vi "Get Travel Reading.vi"(8 "error in (no error)":errorcluster, 11 "ESM303 in":refnum<class "ESM303.lvclass">) -> (0 "error out":errorcluster, 2 "Reading":dbl format="%.4f", 3 "ESM303 out":refnum<class "ESM303.lvclass">)   [LabVIEW 2018, in "ESM303.lvlib" / "ESM303.lvclass"]
uses:
  ESM303.lvclass
  builds/Force Test Stand/Force Test Stand/Force Test Stand.lvlibp/Force Test Stand.lvclass
  C:/Projects/LabVIEW/In-Progress/Jose Rivero-Diaz/builds/Force Test Stand/Force Test Stand/Force Test Stand.lvlibp/Force Test Stand.lvclass
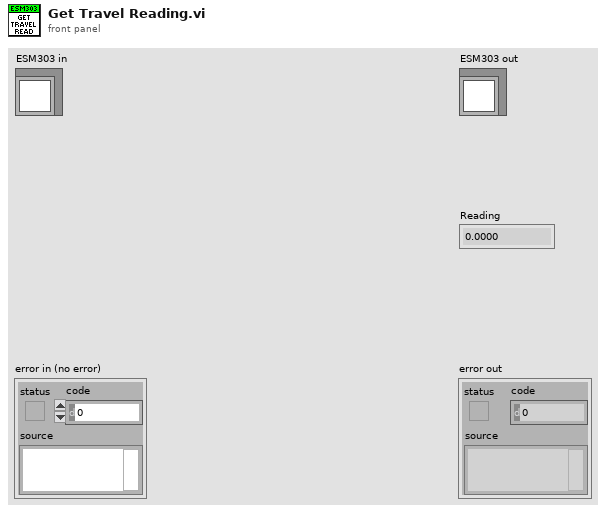
[diagram p1: front panel]
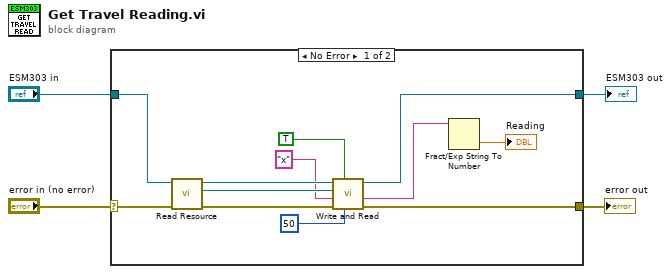
[diagram p0: block diagram]
diagram:
  n1 = case shown="No Error" "error in (no error)" {
    selector: "error in (no error)" -> [w16 w18]
    tunnel: [w6 w18] -> w3
    tunnel: [w8 w17] -> w2
    tunnel: "ESM303 in" -> [w15 w17]
    frame No Error {
      n2 = call "Read Resource.vi"("error in (no error)"=w16, "Force Test Stand in"=w15) -> ("error out"=w12:errorcluster, "Resource"=w13:refnum<visa-resource-name>, "Force Test Stand out"=w14:refnum<class "ESM303.lvclass">)  [unwired: 7 in]
      n3 = call "Write and Read.vi"("Delay Before Read (ms)"=50, "Write & Read"=TRUE, "error in (no error)"=w12, "Command"="x", "VISA Refnum in"=w13, "ESM303 in"=w14) -> ("error out"=w6:errorcluster, "Response"=w7:string, "ESM303 out"=w8:refnum<class "ESM303.lvclass">)  [unwired: 3 in]
      n4 = Fract/Exp String To Number(string=w7) -> (number=→"Reading":dbl)  [unwired: 3 in, 1 out]
    }
    frame Error {
    }
  }
  "error out" <- w3
  "ESM303 out" <- w2
